vi "Lecture 1 example.vi"() -> ()   [LabVIEW 2024]
panel:
  out "Thermometer":dbl(slide) scale=0.0..100.0
  in  "Temp":dbl
  out "LED":bool
  out "z":dbl
  out "y":dbl
  in  "x":dbl
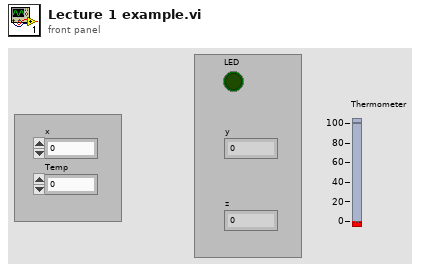
[diagram p1: front panel]
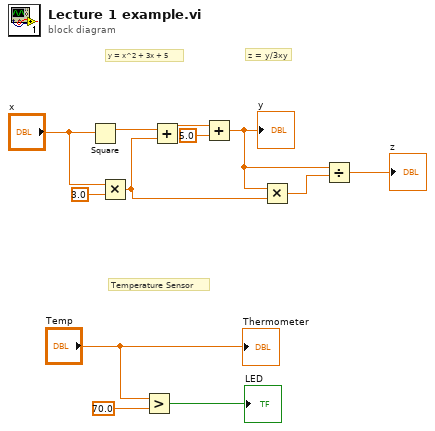
[diagram p0: block diagram]
diagram:
  # "Temperature Sensor"
  # "z = y/3xy"
  # "y = x^2 + 3x + 5"
  n1 = Square(x="x") -> (x^2=w12:dbl)
  n2 = Multiply(x="x", y=3.0) -> (x*y=w7:dbl)
  n3 = Greater?(x="Temp", y=70.0) -> (0:→"LED":bool)
  n4 = Add(x=w12, y=w7) -> (x+y=w9:dbl)
  n5 = Add(x=w9, y=5.0) -> (x+y=w6:dbl)
  "y" <- w6
  n6 = Multiply(x=w6, y=w7) -> (x*y=w5:dbl)
  n7 = Divide(x=w6, y=w5) -> (x/y=→"z":dbl)
  "Thermometer" <- "Temp"
